vi "Simple Scalar FPGA Personality.vi"() -> ()   [LabVIEW 2019]
uses:
  TypeDefs/Simple cluster.ctl
  <vilib>/rvi/Emulation/niFpgaGetClockAttributes.vi
  <vilib>/rvi/Emulation/niFpgaSctlEmulationGetInTimedLoop.vi
  <vilib>/rvi/Emulation/niFpgaEmulationReportErrorSimple.vi
  <vilib>/rvi/Emulation/niFpgaCriticalErrorInLSC.vi
panel:
  in  "Boolean in":bool
  out "Simple cluster out":T1
  in  "Simple cluster in":T1
  in  "Numeric FXP 32/16 in":fxp<+/-,32,16>
  in  "Numeric U8 in":u8
  in  "Numeric U16 in":u16
  in  "Numeric U32 in":u32
  in  "Numeric U64 in":u64
  in  "Numeric I8 in":i8
  in  "Numeric I32 in":i32
  in  "Numeric I64 in":i64
  in  "Numeric SGL in":sgl
  in  "Numeric I16 in":i16
  out "Boolean out":bool
  out "Numeric U8 out":u8
  out "Numeric U16 out":u16
  out "Numeric U32 out":u32
  out "Numeric U64 out":u64
  out "Numeric I8 out":i8
  out "Numeric I32 out":i32
  out "Numeric I64 out":i64
  out "Numeric FXP 32/16 out":fxp<+/-,32,16>
  out "Numeric SGL out":sgl
  out "Numeric I16 out":i16
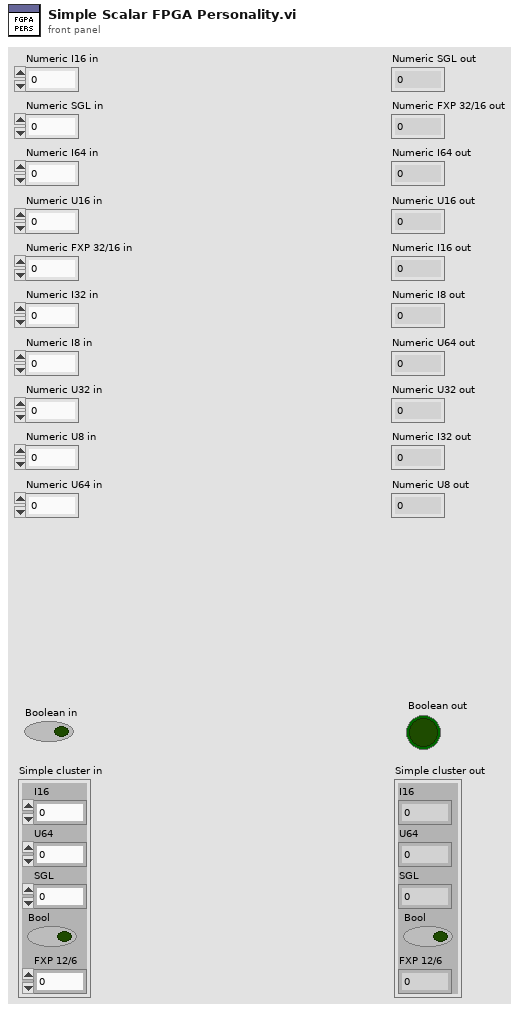
[diagram p1: front panel]
types:
  T1 = typedef "Simple cluster.ctl" = cluster{"I16":i16, "U64":u64, "SGL":sgl, "Bool":bool, "FXP 12/6":fxp<+/-,12,6>}
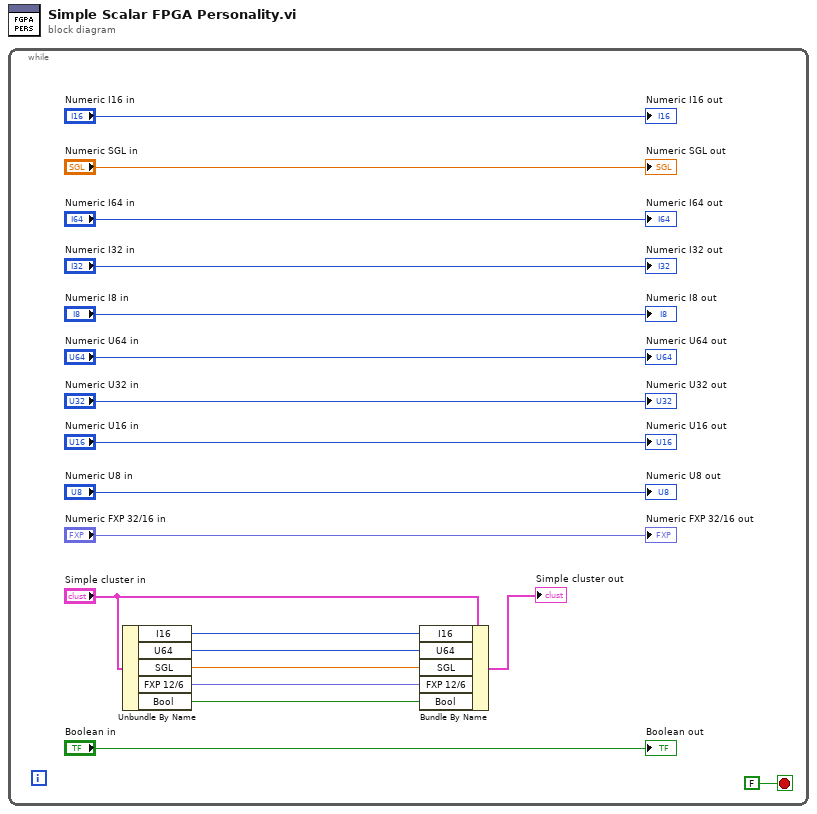
[diagram p0: block diagram]
diagram:
  n1 = while {
    stop <- FALSE stop-if-true
    n2 = Unbundle By Name("Simple cluster in") -> ("I16"=w6:i16, "U64"=w5:u64, "SGL"=w4:sgl, "FXP 12/6"=w3:fxp<+/-,12,6>, "Bool"=w2:bool)
    n3 = Bundle By Name(cluster="Simple cluster in", "I16"=w6, "U64"=w5, "SGL"=w4, "FXP 12/6"=w3, "Bool"=w2) -> (→"Simple cluster out":T1)
    "Numeric I16 out" <- "Numeric I16 in"
    "Numeric SGL out" <- "Numeric SGL in"
    "Numeric FXP 32/16 out" <- "Numeric FXP 32/16 in"
    "Numeric I64 out" <- "Numeric I64 in"
    "Numeric I32 out" <- "Numeric I32 in"
    "Numeric I8 out" <- "Numeric I8 in"
    "Numeric U64 out" <- "Numeric U64 in"
    "Numeric U32 out" <- "Numeric U32 in"
    "Numeric U16 out" <- "Numeric U16 in"
    "Numeric U8 out" <- "Numeric U8 in"
    "Boolean out" <- "Boolean in"
  }
